vi "Keysight DAQ970-Example2.vi"() -> ()   [LabVIEW 2020, in "Keysight DAQ970.lvlib"]
doc: "This Example initializes the driver, reads a few Identity attributes, Reads Monitor Data ,Read Scan Data and checks the instrument error queue. ."
uses:
  Keysight DAQ970.lvlib
panel:
  out "Display Details":string
  out "Info":T1
  out "Simulate":bool
  in  "Simulate":bool=TRUE
  in  "Select ?":bool=TRUE
  in  "Resource String":string="DAQ2"
  in  "Options String":string="DriverSetup= "
  # "Keysight DAQ970 - Example 2"
  # "------------------------------------------------------------------------------------------------------------------------------------------------------------------------------------------------------------------------"
  # "© Keysight Technologies  2020 - 2021"
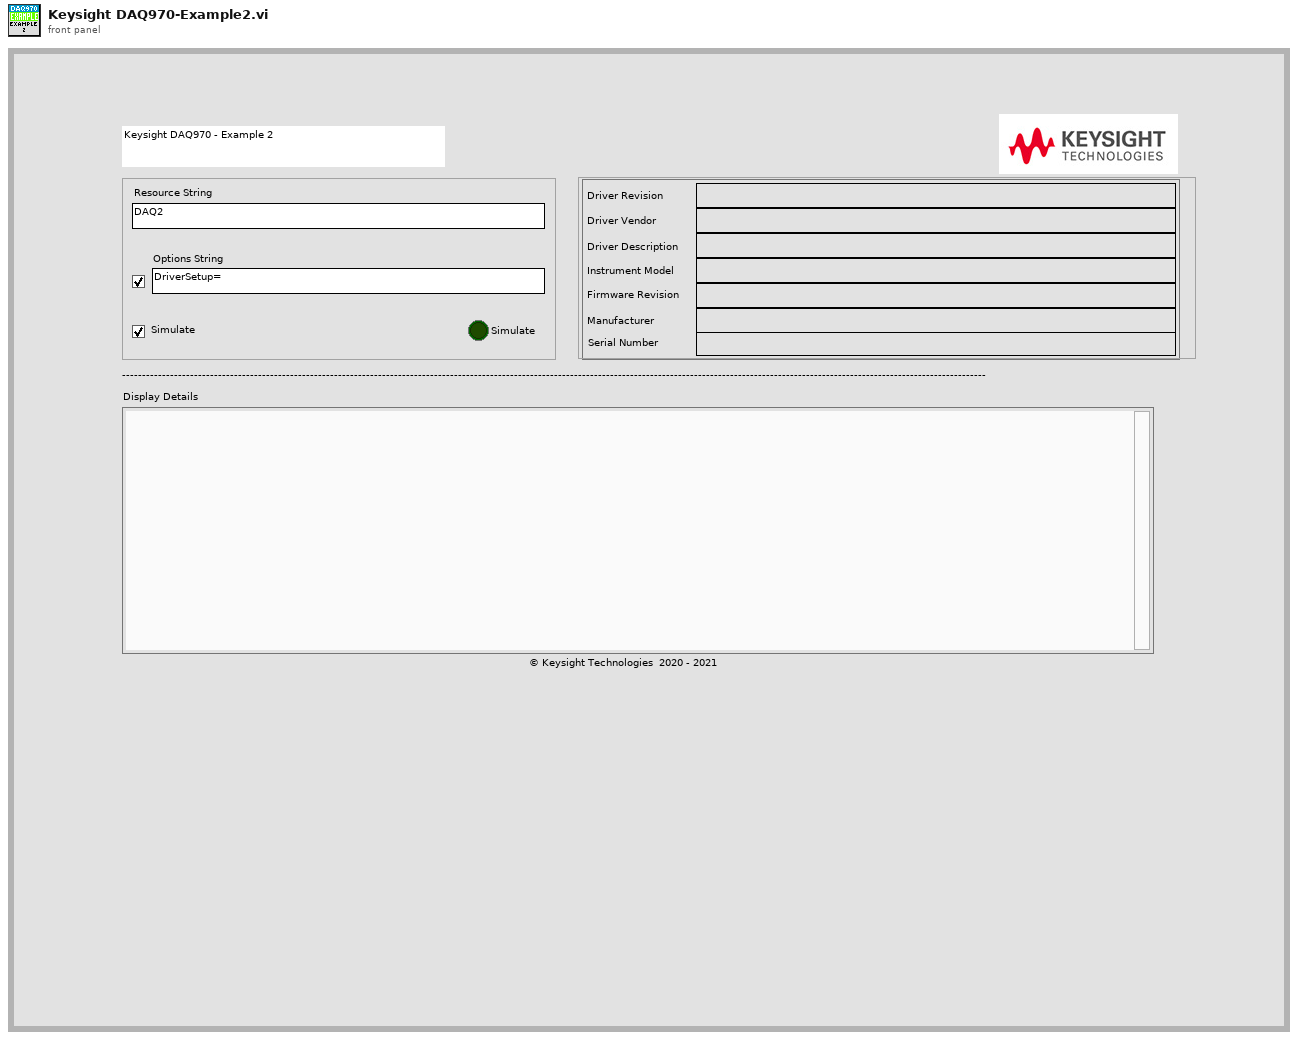
[diagram p1: front panel]
types:
  T1 = cluster{"Driver Revision":string, "Driver Vendor":string, "Driver Description":string, "Instrument Model":string, "Firmware Revision":string, "Instrument Model 2":string, "Firmware Revision 2":string}
  T2 = cluster{"[0]":string, "[1]":string, "[2]":string, "[3]":string, "[4]":string, "[5]":string, "[6]":string}
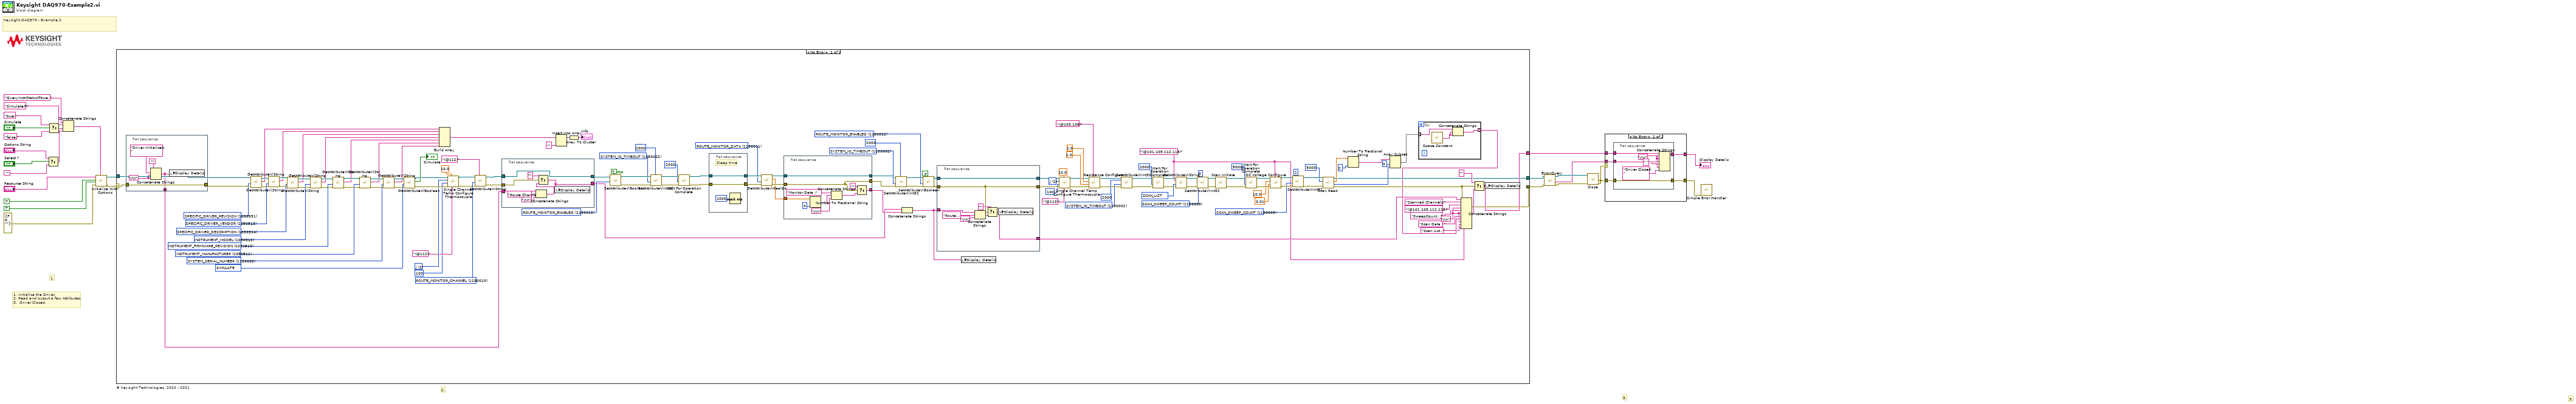
[diagram p0: block diagram]
diagram:
  # "2."
  # "3."
  # "3."
  # "1."
  # "1. Initialize the Driver.\n2. Read and output a few Attributes.\n3.  Driver Closed."
  # "© Keysight Technologies  2020 - 2021"
  # "Keysight DAQ970 - Example 2"
  n1 = Select(t="Options String", s="Select ?", f="") -> (s? t:f=w23:string)
  n2 = Select(t="true,", s="Simulate", f="false,") -> (s? t:f=w25:string)
  n3 = Concatenate Strings("QueryInstrStatus=true, " ("string"), "Simulate=" ("string"), w25, w23) -> (w7:string)
  n4 = call "Initialize With Options.vi"("option string"=w7, "error in (no error)"=errorcluster {"status"=FALSE, "code"=0, "source"=""}, "reset device (Off)"=TRUE, "id query (Off)"=TRUE, "resource string"="Resource String") -> ("error out"=w13:errorcluster, "instrument handle out"=w12:refnum<k15>)  [unwired: 5 in]
  n5 = case shown="No Error" w13 {
    selector: w13 -> [w168 w207]
    tunnel: [w37 w207] -> w3
    tunnel: w12 -> [w139 w206]
    tunnel: [w38 w206] -> w5
    tunnel: [w39 _] -> w15
    frame No Error {
      w27 = "\r\n"
      w51 = u32 1150008 items=["ALARM_MODE"=1150006, "ALARM_SLOPE"=1150007, "FORMAT_TIME_MODE"=1150026, "ROUTE_MONITOR_VIEW"=1150068, "SCAN_CHANNEL_ADVANCE_SOURCE"=1150028, "SCAN_READING_THRESHOLD"=1150031, "SCAN_SINGLE_CHANNEL_SAMPLE_COUNT_PRE_TRIGGER"=1150063, "SCAN_SINGLE_CHANNEL_SAMPLE_COUNT"=1150062, "SCAN_SWEEP_COUNT"=1150008, "SCAN_TRIGGER_OUTPUT_SLOPE"=1150067, "SCAN_TRIGGER_SLOPE"=1150061, "SCAN_TRIGGER_SOURCE"=1150009, "STATUS_ALARM_ENABLE_REGISTER"=1150040, "STATUS_OPERATION_ENABLE_REGISTER"=1150044, "STATUS_QUESTIONABLE_ENABLE_REGISTER"=1150045, "STATUS_SERVICE_REQUEST_ENABLE_REGISTER"=1150047, "STATUS_STANDARD_EVENT_ENABLE_REGISTER"=1150046, "SYSTEM_AUTOCALIBRATION_MONTHLY_INTERVAL_DAY"=1150049, "SYSTEM_AUTOCALIBRATION_OCCURENCE_INTERVAL"=1150048, "SYSTEM_AUTOCALIBRATION_WEEKLY_INTERVAL_DAY"=1150050, "SYSTEM_IO_TIMEOUT"=1150002, "SYSTEM_TRACING_LEVEL"=1150043, "USB_MEMORY_COLUMN_HEADER"=1150054, "USB_MEMORY_COLUMN_SEPARATOR"=1150035, "USB_MEMORY_ROW_LIMIT_COUNT"=1150055] ("AttributeID")
      w128 = 2 items=["b", "g", "j", "k", "n", "r", "s", "t", "def"] ("Type (b)")
      w63 = u32 1150008 items=["ALARM_MODE"=1150006, "ALARM_SLOPE"=1150007, "FORMAT_TIME_MODE"=1150026, "ROUTE_MONITOR_VIEW"=1150068, "SCAN_CHANNEL_ADVANCE_SOURCE"=1150028, "SCAN_READING_THRESHOLD"=1150031, "SCAN_SINGLE_CHANNEL_SAMPLE_COUNT_PRE_TRIGGER"=1150063, "SCAN_SINGLE_CHANNEL_SAMPLE_COUNT"=1150062, "SCAN_SWEEP_COUNT"=1150008, "SCAN_TRIGGER_OUTPUT_SLOPE"=1150067, "SCAN_TRIGGER_SLOPE"=1150061, "SCAN_TRIGGER_SOURCE"=1150009, "STATUS_ALARM_ENABLE_REGISTER"=1150040, "STATUS_OPERATION_ENABLE_REGISTER"=1150044, "STATUS_QUESTIONABLE_ENABLE_REGISTER"=1150045, "STATUS_SERVICE_REQUEST_ENABLE_REGISTER"=1150047, "STATUS_STANDARD_EVENT_ENABLE_REGISTER"=1150046, "SYSTEM_AUTOCALIBRATION_MONTHLY_INTERVAL_DAY"=1150049, "SYSTEM_AUTOCALIBRATION_OCCURENCE_INTERVAL"=1150048, "SYSTEM_AUTOCALIBRATION_WEEKLY_INTERVAL_DAY"=1150050, "SYSTEM_IO_TIMEOUT"=1150002, "SYSTEM_TRACING_LEVEL"=1150043, "USB_MEMORY_COLUMN_HEADER"=1150054, "USB_MEMORY_COLUMN_SEPARATOR"=1150035, "USB_MEMORY_ROW_LIMIT_COUNT"=1150055] ("AttributeID")
      w76 = u32 1150002 items=["ALARM_MODE"=1150006, "ALARM_SLOPE"=1150007, "FORMAT_TIME_MODE"=1150026, "ROUTE_MONITOR_VIEW"=1150068, "SCAN_CHANNEL_ADVANCE_SOURCE"=1150028, "SCAN_READING_THRESHOLD"=1150031, "SCAN_SINGLE_CHANNEL_SAMPLE_COUNT_PRE_TRIGGER"=1150063, "SCAN_SINGLE_CHANNEL_SAMPLE_COUNT"=1150062, "SCAN_SWEEP_COUNT"=1150008, "SCAN_TRIGGER_OUTPUT_SLOPE"=1150067, "SCAN_TRIGGER_SLOPE"=1150061, "SCAN_TRIGGER_SOURCE"=1150009, "STATUS_ALARM_ENABLE_REGISTER"=1150040, "STATUS_OPERATION_ENABLE_REGISTER"=1150044, "STATUS_QUESTIONABLE_ENABLE_REGISTER"=1150045, "STATUS_SERVICE_REQUEST_ENABLE_REGISTER"=1150047, "STATUS_STANDARD_EVENT_ENABLE_REGISTER"=1150046, "SYSTEM_AUTOCALIBRATION_MONTHLY_INTERVAL_DAY"=1150049, "SYSTEM_AUTOCALIBRATION_OCCURENCE_INTERVAL"=1150048, "SYSTEM_AUTOCALIBRATION_WEEKLY_INTERVAL_DAY"=1150050, "SYSTEM_IO_TIMEOUT"=1150002, "SYSTEM_TRACING_LEVEL"=1150043, "USB_MEMORY_COLUMN_HEADER"=1150054, "USB_MEMORY_COLUMN_SEPARATOR"=1150035, "USB_MEMORY_ROW_LIMIT_COUNT"=1150055] ("AttributeID")
      w81 = 2 items=["B", "E", "J", "K", "N", "r", "S", "T"] ("ThermocoupleType (B)")
      w88 = u32 1150012 items=["DISPLAY_ENABLED"=1150016, "FORMAT_ALARM_ENABLED"=1150023, "FORMAT_CHANNEL_ENABLED"=1150024, "FORMAT_TIME_ENABLED"=1150025, "FORMAT_UNITS_ENABLED"=1150027, "ROUTE_MONITOR_ENABLED"=1150012, "SIMULATE"=1050005, "SYSTEM_DMM_ENABLED"=1150018, "SYSTEM_INSTRUMENT_STATE_POWER_ON_RECALL_ENABLED"=1150033, "SYSTEM_LXI_IDENTIFY_ENABLED"=1150032, "SYSTEM_TRACING_ENABLED"=1150041, "USB_MEMORY_LOGGING_ENABLED"=1150034, "USB_MEMORY_MEASUREMENT_DATA_AUTO_SAVE_ENABLED"=1150057, "USB_MEMORY_RECALL_AUTO_ENABLED"=1150052, "USB_MEMORY_ROW_LIMIT_ENABLED"=1150036] ("AttributeID")
      w93 = u32 1150002 items=["ALARM_MODE"=1150006, "ALARM_SLOPE"=1150007, "FORMAT_TIME_MODE"=1150026, "ROUTE_MONITOR_VIEW"=1150068, "SCAN_CHANNEL_ADVANCE_SOURCE"=1150028, "SCAN_READING_THRESHOLD"=1150031, "SCAN_SINGLE_CHANNEL_SAMPLE_COUNT_PRE_TRIGGER"=1150063, "SCAN_SINGLE_CHANNEL_SAMPLE_COUNT"=1150062, "SCAN_SWEEP_COUNT"=1150008, "SCAN_TRIGGER_OUTPUT_SLOPE"=1150067, "SCAN_TRIGGER_SLOPE"=1150061, "SCAN_TRIGGER_SOURCE"=1150009, "STATUS_ALARM_ENABLE_REGISTER"=1150040, "STATUS_OPERATION_ENABLE_REGISTER"=1150044, "STATUS_QUESTIONABLE_ENABLE_REGISTER"=1150045, "STATUS_SERVICE_REQUEST_ENABLE_REGISTER"=1150047, "STATUS_STANDARD_EVENT_ENABLE_REGISTER"=1150046, "SYSTEM_AUTOCALIBRATION_MONTHLY_INTERVAL_DAY"=1150049, "SYSTEM_AUTOCALIBRATION_OCCURENCE_INTERVAL"=1150048, "SYSTEM_AUTOCALIBRATION_WEEKLY_INTERVAL_DAY"=1150050, "SYSTEM_IO_TIMEOUT"=1150002, "SYSTEM_TRACING_LEVEL"=1150043, "USB_MEMORY_COLUMN_HEADER"=1150054, "USB_MEMORY_COLUMN_SEPARATOR"=1150035, "USB_MEMORY_ROW_LIMIT_COUNT"=1150055] ("AttributeID")
      w98 = u32 1150011 items=["ROUTE_MONITOR_DATA"=1150011, "ROUTE_MONITOR_FULL_DATA"=1150069, "SCAN_SINGLE_CHANNEL_SAMPLE_INTERVAL"=1150064, "SCAN_TIMER_INTERVAL"=1150029, "SCAN_TRIGGER_DELAY"=1150059, "SCAN_TRIGGER_LEVEL"=1150060, "SYSTEM_LINE_FREQUENCY"=1150037] ("AttributeID")
      w107 = u32 1150002 items=["ALARM_MODE"=1150006, "ALARM_SLOPE"=1150007, "FORMAT_TIME_MODE"=1150026, "ROUTE_MONITOR_VIEW"=1150068, "SCAN_CHANNEL_ADVANCE_SOURCE"=1150028, "SCAN_READING_THRESHOLD"=1150031, "SCAN_SINGLE_CHANNEL_SAMPLE_COUNT_PRE_TRIGGER"=1150063, "SCAN_SINGLE_CHANNEL_SAMPLE_COUNT"=1150062, "SCAN_SWEEP_COUNT"=1150008, "SCAN_TRIGGER_OUTPUT_SLOPE"=1150067, "SCAN_TRIGGER_SLOPE"=1150061, "SCAN_TRIGGER_SOURCE"=1150009, "STATUS_ALARM_ENABLE_REGISTER"=1150040, "STATUS_OPERATION_ENABLE_REGISTER"=1150044, "STATUS_QUESTIONABLE_ENABLE_REGISTER"=1150045, "STATUS_SERVICE_REQUEST_ENABLE_REGISTER"=1150047, "STATUS_STANDARD_EVENT_ENABLE_REGISTER"=1150046, "SYSTEM_AUTOCALIBRATION_MONTHLY_INTERVAL_DAY"=1150049, "SYSTEM_AUTOCALIBRATION_OCCURENCE_INTERVAL"=1150048, "SYSTEM_AUTOCALIBRATION_WEEKLY_INTERVAL_DAY"=1150050, "SYSTEM_IO_TIMEOUT"=1150002, "SYSTEM_TRACING_LEVEL"=1150043, "USB_MEMORY_COLUMN_HEADER"=1150054, "USB_MEMORY_COLUMN_SEPARATOR"=1150035, "USB_MEMORY_ROW_LIMIT_COUNT"=1150055] ("AttributeID")
      w117 = u32 1150010 items=["CALIBRATION_MESSAGE"=1150015, "DISPLAY_TEXT"=1150017, "ROUTE_MONITOR_CHANNEL"=1150010, "SCAN_LIST"=1150004, "SYSTEM_DATE"=1150020, "SYSTEM_TIME"=1150021, "SYSTEM_TRACING_FILE_NAME"=1150042, "USB_MEMORY_DATA_FILE"=1150056, "USB_MEMORY_MEASUREMENTS_DATA_AUTO_SAVE_FILE"=1150058, "USB_MEMORY_SELECT_RECALL_AUTO_FILE"=1150053] ("AttributeID")
      w120 = u32 1150012 items=["DISPLAY_ENABLED"=1150016, "FORMAT_ALARM_ENABLED"=1150023, "FORMAT_CHANNEL_ENABLED"=1150024, "FORMAT_TIME_ENABLED"=1150025, "FORMAT_UNITS_ENABLED"=1150027, "ROUTE_MONITOR_ENABLED"=1150012, "SIMULATE"=1050005, "SYSTEM_DMM_ENABLED"=1150018, "SYSTEM_INSTRUMENT_STATE_POWER_ON_RECALL_ENABLED"=1150033, "SYSTEM_LXI_IDENTIFY_ENABLED"=1150032, "SYSTEM_TRACING_ENABLED"=1150041, "USB_MEMORY_LOGGING_ENABLED"=1150034, "USB_MEMORY_MEASUREMENT_DATA_AUTO_SAVE_ENABLED"=1150057, "USB_MEMORY_RECALL_AUTO_ENABLED"=1150052, "USB_MEMORY_ROW_LIMIT_ENABLED"=1150036] ("AttributeID")
      w121 = u32 1150004 items=["CALIBRATION_MESSAGE"=1150015, "DISPLAY_TEXT"=1150017, "ROUTE_MONITOR_CHANNEL"=1150010, "SCAN_LIST"=1150004, "SYSTEM_DATE"=1150020, "SYSTEM_TIME"=1150021, "SYSTEM_TRACING_FILE_NAME"=1150042, "USB_MEMORY_DATA_FILE"=1150056, "USB_MEMORY_MEASUREMENTS_DATA_AUTO_SAVE_FILE"=1150058, "USB_MEMORY_SELECT_RECALL_AUTO_FILE"=1150053] ("AttributeID")
      w162 = u32 1050005 items=["DISPLAY_ENABLED"=1150016, "FORMAT_ALARM_ENABLED"=1150023, "FORMAT_CHANNEL_ENABLED"=1150024, "FORMAT_TIME_ENABLED"=1150025, "FORMAT_UNITS_ENABLED"=1150027, "ROUTE_MONITOR_ENABLED"=1150012, "SIMULATE"=1050005, "SYSTEM_AUTOCALIBRATION_GET_ALL_MODULE_STATE"=1150051, "SYSTEM_DMM_ENABLED"=1150018, "SYSTEM_DMM_INSTALLED"=1150019, "SYSTEM_INSTRUMENT_STATE_POWER_ON_RECALL_ENABLED"=1150033, "SYSTEM_LXI_IDENTIFY_ENABLED"=1150032, "SYSTEM_TRACING_ENABLED"=1150041, "USB_MEMORY_LOGGING_ENABLED"=1150034, "USB_MEMORY_MEASUREMENT_DATA_AUTO_SAVE_ENABLED"=1150057, "USB_MEMORY_RECALL_AUTO_ENABLED"=1150052, "USB_MEMORY_ROW_LIMIT_ENABLED"=1150036] ("AttributeID")
      w161 = u32 1150003 items=["CALIBRATION_DATE"=1150065, "CALIBRATION_MESSAGE"=1150015, "CALIBRATION_TIME"=1150066, "DISPLAY_TEXT"=1150017, "DRIVER_SETUP"=1050007, "GROUP_CAPABILITIES"=1050401, "INSTRUMENT_FIRMWARE_REVISION"=1050510, "INSTRUMENT_MANUFACTURER"=1050511, "INSTRUMENT_MODEL"=1050512, "IO_RESOURCE_DESCRIPTOR"=1050304, "LOGICAL_NAME"=1050305, "ROUTE_MONITOR_CHANNEL"=1150010, "SCAN_LIST"=1150004, "SCAN_STARTTIME"=1150022, "SPECIFIC_DRIVER_DESCRIPTION"=1050514, "SPECIFIC_DRIVER_PREFIX"=1050302, "SPECIFIC_DRIVER_REVISION"=1050551, "SPECIFIC_DRIVER_VENDOR"=1050513, "SUPPORTED_INSTRUMENT_MODELS"=1050327, "SYSTEM_DATE"=1150020, "SYSTEM_SERIAL_NUMBER"=1150003, "SYSTEM_TIME"=1150021, "SYSTEM_TRACING_FILE_NAME"=1150042, "USB_MEMORY_DATA_FILE"=1150056, "USB_MEMORY_MEASUREMENTS_DATA_AUTO_SAVE_FILE"=1150058, "USB_MEMORY_SELECT_RECALL_AUTO_FILE"=1150053] ("AttributeID")
      w160 = u32 1050511 items=["CALIBRATION_DATE"=1150065, "CALIBRATION_MESSAGE"=1150015, "CALIBRATION_TIME"=1150066, "DISPLAY_TEXT"=1150017, "DRIVER_SETUP"=1050007, "GROUP_CAPABILITIES"=1050401, "INSTRUMENT_FIRMWARE_REVISION"=1050510, "INSTRUMENT_MANUFACTURER"=1050511, "INSTRUMENT_MODEL"=1050512, "IO_RESOURCE_DESCRIPTOR"=1050304, "LOGICAL_NAME"=1050305, "ROUTE_MONITOR_CHANNEL"=1150010, "SCAN_LIST"=1150004, "SCAN_STARTTIME"=1150022, "SPECIFIC_DRIVER_DESCRIPTION"=1050514, "SPECIFIC_DRIVER_PREFIX"=1050302, "SPECIFIC_DRIVER_REVISION"=1050551, "SPECIFIC_DRIVER_VENDOR"=1050513, "SUPPORTED_INSTRUMENT_MODELS"=1050327, "SYSTEM_DATE"=1150020, "SYSTEM_SERIAL_NUMBER"=1150003, "SYSTEM_TIME"=1150021, "SYSTEM_TRACING_FILE_NAME"=1150042, "USB_MEMORY_DATA_FILE"=1150056, "USB_MEMORY_MEASUREMENTS_DATA_AUTO_SAVE_FILE"=1150058, "USB_MEMORY_SELECT_RECALL_AUTO_FILE"=1150053] ("AttributeID")
      w159 = u32 1050510 items=["CALIBRATION_DATE"=1150065, "CALIBRATION_MESSAGE"=1150015, "CALIBRATION_TIME"=1150066, "DISPLAY_TEXT"=1150017, "DRIVER_SETUP"=1050007, "GROUP_CAPABILITIES"=1050401, "INSTRUMENT_FIRMWARE_REVISION"=1050510, "INSTRUMENT_MANUFACTURER"=1050511, "INSTRUMENT_MODEL"=1050512, "IO_RESOURCE_DESCRIPTOR"=1050304, "LOGICAL_NAME"=1050305, "ROUTE_MONITOR_CHANNEL"=1150010, "SCAN_LIST"=1150004, "SCAN_STARTTIME"=1150022, "SPECIFIC_DRIVER_DESCRIPTION"=1050514, "SPECIFIC_DRIVER_PREFIX"=1050302, "SPECIFIC_DRIVER_REVISION"=1050551, "SPECIFIC_DRIVER_VENDOR"=1050513, "SUPPORTED_INSTRUMENT_MODELS"=1050327, "SYSTEM_DATE"=1150020, "SYSTEM_SERIAL_NUMBER"=1150003, "SYSTEM_TIME"=1150021, "SYSTEM_TRACING_FILE_NAME"=1150042, "USB_MEMORY_DATA_FILE"=1150056, "USB_MEMORY_MEASUREMENTS_DATA_AUTO_SAVE_FILE"=1150058, "USB_MEMORY_SELECT_RECALL_AUTO_FILE"=1150053] ("AttributeID")
      w158 = u32 1050512 items=["CALIBRATION_DATE"=1150065, "CALIBRATION_MESSAGE"=1150015, "CALIBRATION_TIME"=1150066, "DISPLAY_TEXT"=1150017, "DRIVER_SETUP"=1050007, "GROUP_CAPABILITIES"=1050401, "INSTRUMENT_FIRMWARE_REVISION"=1050510, "INSTRUMENT_MANUFACTURER"=1050511, "INSTRUMENT_MODEL"=1050512, "IO_RESOURCE_DESCRIPTOR"=1050304, "LOGICAL_NAME"=1050305, "ROUTE_MONITOR_CHANNEL"=1150010, "SCAN_LIST"=1150004, "SCAN_STARTTIME"=1150022, "SPECIFIC_DRIVER_DESCRIPTION"=1050514, "SPECIFIC_DRIVER_PREFIX"=1050302, "SPECIFIC_DRIVER_REVISION"=1050551, "SPECIFIC_DRIVER_VENDOR"=1050513, "SUPPORTED_INSTRUMENT_MODELS"=1050327, "SYSTEM_DATE"=1150020, "SYSTEM_SERIAL_NUMBER"=1150003, "SYSTEM_TIME"=1150021, "SYSTEM_TRACING_FILE_NAME"=1150042, "USB_MEMORY_DATA_FILE"=1150056, "USB_MEMORY_MEASUREMENTS_DATA_AUTO_SAVE_FILE"=1150058, "USB_MEMORY_SELECT_RECALL_AUTO_FILE"=1150053] ("AttributeID")
      w157 = u32 1050514 items=["CALIBRATION_DATE"=1150065, "CALIBRATION_MESSAGE"=1150015, "CALIBRATION_TIME"=1150066, "DISPLAY_TEXT"=1150017, "DRIVER_SETUP"=1050007, "GROUP_CAPABILITIES"=1050401, "INSTRUMENT_FIRMWARE_REVISION"=1050510, "INSTRUMENT_MANUFACTURER"=1050511, "INSTRUMENT_MODEL"=1050512, "IO_RESOURCE_DESCRIPTOR"=1050304, "LOGICAL_NAME"=1050305, "ROUTE_MONITOR_CHANNEL"=1150010, "SCAN_LIST"=1150004, "SCAN_STARTTIME"=1150022, "SPECIFIC_DRIVER_DESCRIPTION"=1050514, "SPECIFIC_DRIVER_PREFIX"=1050302, "SPECIFIC_DRIVER_REVISION"=1050551, "SPECIFIC_DRIVER_VENDOR"=1050513, "SUPPORTED_INSTRUMENT_MODELS"=1050327, "SYSTEM_DATE"=1150020, "SYSTEM_SERIAL_NUMBER"=1150003, "SYSTEM_TIME"=1150021, "SYSTEM_TRACING_FILE_NAME"=1150042, "USB_MEMORY_DATA_FILE"=1150056, "USB_MEMORY_MEASUREMENTS_DATA_AUTO_SAVE_FILE"=1150058, "USB_MEMORY_SELECT_RECALL_AUTO_FILE"=1150053] ("AttributeID")
      w156 = u32 1050513 items=["CALIBRATION_DATE"=1150065, "CALIBRATION_MESSAGE"=1150015, "CALIBRATION_TIME"=1150066, "DISPLAY_TEXT"=1150017, "DRIVER_SETUP"=1050007, "GROUP_CAPABILITIES"=1050401, "INSTRUMENT_FIRMWARE_REVISION"=1050510, "INSTRUMENT_MANUFACTURER"=1050511, "INSTRUMENT_MODEL"=1050512, "IO_RESOURCE_DESCRIPTOR"=1050304, "LOGICAL_NAME"=1050305, "ROUTE_MONITOR_CHANNEL"=1150010, "SCAN_LIST"=1150004, "SCAN_STARTTIME"=1150022, "SPECIFIC_DRIVER_DESCRIPTION"=1050514, "SPECIFIC_DRIVER_PREFIX"=1050302, "SPECIFIC_DRIVER_REVISION"=1050551, "SPECIFIC_DRIVER_VENDOR"=1050513, "SUPPORTED_INSTRUMENT_MODELS"=1050327, "SYSTEM_DATE"=1150020, "SYSTEM_SERIAL_NUMBER"=1150003, "SYSTEM_TIME"=1150021, "SYSTEM_TRACING_FILE_NAME"=1150042, "USB_MEMORY_DATA_FILE"=1150056, "USB_MEMORY_MEASUREMENTS_DATA_AUTO_SAVE_FILE"=1150058, "USB_MEMORY_SELECT_RECALL_AUTO_FILE"=1150053] ("AttributeID")
      w155 = u32 1050551 items=["CALIBRATION_DATE"=1150065, "CALIBRATION_MESSAGE"=1150015, "CALIBRATION_TIME"=1150066, "DISPLAY_TEXT"=1150017, "DRIVER_SETUP"=1050007, "GROUP_CAPABILITIES"=1050401, "INSTRUMENT_FIRMWARE_REVISION"=1050510, "INSTRUMENT_MANUFACTURER"=1050511, "INSTRUMENT_MODEL"=1050512, "IO_RESOURCE_DESCRIPTOR"=1050304, "LOGICAL_NAME"=1050305, "ROUTE_MONITOR_CHANNEL"=1150010, "SCAN_LIST"=1150004, "SCAN_STARTTIME"=1150022, "SPECIFIC_DRIVER_DESCRIPTION"=1050514, "SPECIFIC_DRIVER_PREFIX"=1050302, "SPECIFIC_DRIVER_REVISION"=1050551, "SPECIFIC_DRIVER_VENDOR"=1050513, "SUPPORTED_INSTRUMENT_MODELS"=1050327, "SYSTEM_DATE"=1150020, "SYSTEM_SERIAL_NUMBER"=1150003, "SYSTEM_TIME"=1150021, "SYSTEM_TRACING_FILE_NAME"=1150042, "USB_MEMORY_DATA_FILE"=1150056, "USB_MEMORY_MEASUREMENTS_DATA_AUTO_SAVE_FILE"=1150058, "USB_MEMORY_SELECT_RECALL_AUTO_FILE"=1150053] ("AttributeID")
      w29 = "(@101,105,112,113)" ("AttributeValue")
      n6 = flat-sequence {
        tunnel: w168 -> [w205]
        tunnel: [w205] -> w138
        tunnel: [w201] -> w114
        frame #0 {
          w202 = "\r\n"
          n7 = Concatenate Strings("", "Driver Initialized.", w202, w202) -> (w201:string)
          n8 = local write "Display Details"(w201) -> ()
        }
      }
      n9 = call "GetAttributeViString.vi"("error in (no error)"=w138, "AttributeID"=w155, "instrument handle"=w139) -> ("error out"=w141:errorcluster, "AttributeValue"=w137:string, "instrument handle out"=w142:refnum<k15>)  [unwired: 6 in]
      n10 = call "GetAttributeViString.vi"("error in (no error)"=w141, "AttributeID"=w156, "instrument handle"=w142) -> ("error out"=w143:errorcluster, "AttributeValue"=w136:string, "instrument handle out"=w144:refnum<k15>)  [unwired: 6 in]
      n11 = call "GetAttributeViString.vi"("error in (no error)"=w143, "AttributeID"=w157, "instrument handle"=w144) -> ("error out"=w146:errorcluster, "AttributeValue"=w135:string, "instrument handle out"=w145:refnum<k15>)  [unwired: 6 in]
      n12 = call "GetAttributeViString.vi"("error in (no error)"=w146, "AttributeID"=w158, "instrument handle"=w145) -> ("error out"=w147:errorcluster, "AttributeValue"=w134:string, "instrument handle out"=w148:refnum<k15>)  [unwired: 6 in]
      n13 = call "GetAttributeViString.vi"("error in (no error)"=w147, "AttributeID"=w159, "instrument handle"=w148) -> ("error out"=w149:errorcluster, "AttributeValue"=w133:string, "instrument handle out"=w150:refnum<k15>)  [unwired: 6 in]
      n14 = call "GetAttributeViString.vi"("error in (no error)"=w149, "AttributeID"=w160, "instrument handle"=w150) -> ("error out"=w152:errorcluster, "AttributeValue"=w132:string, "instrument handle out"=w151:refnum<k15>)  [unwired: 6 in]
      n15 = call "GetAttributeViString.vi"("error in (no error)"=w152, "AttributeID"=w161, "instrument handle"=w151) -> ("error out"=w154:errorcluster, "AttributeValue"=w131:string, "instrument handle out"=w153:refnum<k15>)  [unwired: 6 in]
      n16 = call "GetAttributeViBoolean.vi"("error in (no error)"=w154, "AttributeID"=w162, "instrument handle"=w153) -> ("error out"=w130:errorcluster, "AttributeValue"=→"Simulate":bool, "instrument handle out"=w129:refnum<k15>)  [unwired: 6 in]
      n17 = Build Array(w137, w136, w135, w134, w133, w132, w131) -> (w165:string[])
      n18 = call "Single Channel Temp Configure Thermocouple.vi"("Channel"="(@112)" ("ChannelList"), "SampTime"=10.0 ("Sample Time"), "error in (no error)"=w130, "SampCount"=100, "ThermocoupleType (B)"=w128, "instrument handle"=w129) -> ("error out"=w116:errorcluster, "instrument handle out"=w118:refnum<k15>)  [unwired: 4 in]
      n19 = call "SetAttributeViString.vi"("AttributeValue"="(@112)", "error in (no error)"=w116, "AttributeID"=w117, "instrument handle"=w118) -> ("error out"=w113:errorcluster, "instrument handle out"=w112:refnum<k15>)  [unwired: 6 in]
      n20 = flat-sequence {
        tunnel: w114 -> [w192]
        tunnel: w113 -> [w188]
        tunnel: [w186] -> w99
        tunnel: [w191] -> w111
        tunnel: w112 -> [w191]
        frame #0 {
          n21 = Concatenate Strings(w192, "Route Channel Monitoring Enabled !!!", "\r\n") -> (w187:string)
          n22 = Select(t="", s=w188, f=w187) -> (s? t:f=w186:string)
          n23 = local write "Display Details"(w186) -> ()
        }
      }
      n24 = Insert Into Array(array=w165, new element="" ("new element/subarray")) -> (w166:string[])  [unwired: 1 in]
      n25 = Array To Cluster(array=w166) -> (cluster=→"Info":T2)
      n26 = call "SetAttributeViBoolean.vi"("AttributeValue (Off)"=TRUE, "AttributeID"=w120, "instrument handle"=w111) -> ("error out"=w109:errorcluster, "instrument handle out"=w110:refnum<k15>)  [unwired: 7 in]
      n27 = call "SetAttributeViInt32.vi"("AttributeValue"=2000, "error in (no error)"=w109, "AttributeID"=w107, "instrument handle"=w110) -> ("error out"=w105:errorcluster, "instrument handle out"=w106:refnum<k15>)  [unwired: 6 in]
      n28 = call "Wait For Operation Complete.vi"("error in (no error)"=w105, "MaxTimeMilliseconds"=2000, "instrument handle"=w106) -> ("error out"=w102:errorcluster, "instrument handle out"=w103:refnum<k15>)  [unwired: 7 in]
      n29 = flat-sequence {
        tunnel: [w183] -> w101
        tunnel: w103 -> [w183]
        tunnel: [w182] -> w100
        tunnel: w102 -> [w182]
        frame #0 {
          # "Sleep time"
          n30 = Wait (ms)(milliseconds to wait=u32 1000) -> ()  [unwired: 1 out]
        }
      }
      n31 = call "GetAttributeViReal64.vi"("error in (no error)"=w100, "AttributeID"=w98, "instrument handle"=w101) -> ("error out"=w97:errorcluster, "AttributeValue"=w36:dbl, "instrument handle out"=w96:refnum<k15>)  [unwired: 6 in]
      n32 = flat-sequence {
        tunnel: w97 -> [w174]
        tunnel: [w176] -> w92
        tunnel: w96 -> [w176]
        tunnel: [w175] -> w95
        tunnel: [w174] -> w91
        tunnel: w36 -> [w173]
        frame #0 {
          n33 = Number To Fractional String(number=w173, precision (6)=i16 0) -> (F-format string=w180:string)  [unwired: 2 in]
          n34 = Concatenate Strings("Monitor Data :", w180, "\r\n") -> (w179:string)
          n35 = Select(t="", s=w174, f=w179) -> (s? t:f=w175:string)
        }
      }
      n36 = call "SetAttributeViInt32.vi"("AttributeValue"=2000, "error in (no error)"=w91, "AttributeID"=w93, "instrument handle"=w92) -> ("error out"=w89:errorcluster, "instrument handle out"=w90:refnum<k15>)  [unwired: 6 in]
      n37 = Concatenate Strings(w99, w95) -> (w164:string)
      n38 = call "SetAttributeViBoolean.vi"("AttributeValue (Off)"=FALSE, "error in (no error)"=w89, "AttributeID"=w88, "instrument handle"=w90) -> ("error out"=w85:errorcluster, "instrument handle out"=w86:refnum<k15>)  [unwired: 6 in]
      n39 = flat-sequence {
        tunnel: [w193] -> w83
        tunnel: w164 -> [w200]
        tunnel: [w196] -> w40
        tunnel: [w194] -> w84
        tunnel: w86 -> [w194]
        tunnel: w85 -> [w193]
        frame #0 {
          n40 = Concatenate Strings(w200, "Route Channel Monitoring Disabled !!!", "\r\n") -> (w197:string)
          n41 = Select(t="", s=w193, f=w197) -> (s? t:f=w196:string)
          n42 = local write "Display Details"(w196) -> ()
        }
      }
      n43 = local write "Display Details"(w164) -> ()
      n44 = call "Single Channel Temp Configure Thermocouple.vi"("Channel"="(@113)", "SampTime"=10.0, "error in (no error)"=w83, "SampCount"=100, "ThermocoupleType (B)"=w81, "instrument handle"=w84) -> ("error out"=w77:errorcluster, "instrument handle out"=w78:refnum<k15>)  [unwired: 4 in]
      n45 = call "Resistance Configure.vi"("ChannelList"="(@103,108)", "error in (no error)"=w77, "Resolution"=1.0, "Range"=1.0, "instrument handle"=w78) -> ("error out"=w74:errorcluster, "instrument handle out"=w73:refnum<k15>)  [unwired: 5 in]
      n46 = call "SetAttributeViInt32.vi"("AttributeValue"=2000, "error in (no error)"=w74, "AttributeID"=w76, "instrument handle"=w73) -> ("error out"=w70:errorcluster, "instrument handle out"=w71:refnum<k15>)  [unwired: 6 in]
      n47 = call "Wait For Operation Complete.vi"("error in (no error)"=w70, "MaxTimeMilliseconds"=2000, "instrument handle"=w71) -> ("error out"=w69:errorcluster, "instrument handle out"=w68:refnum<k15>)  [unwired: 7 in]
      n48 = call "SetAttributeViString.vi"("AttributeValue"=w29, "error in (no error)"=w69, "AttributeID"=w121, "instrument handle"=w68) -> ("error out"=w66:errorcluster, "instrument handle out"=w67:refnum<k15>)  [unwired: 6 in]
      n49 = call "SetAttributeViInt32.vi"("AttributeValue"=5, "error in (no error)"=w66, "AttributeID"=w63, "instrument handle"=w67) -> ("error out"=w64:errorcluster, "instrument handle out"=w65:refnum<k15>)  [unwired: 6 in]
      n50 = call "Scan Initiate.vi"("error in (no error)"=w64, "instrument handle"=w65) -> ("error out"=w59:errorcluster, "instrument handle out"=w60:refnum<k15>)  [unwired: 8 in]
      n51 = call "Wait For Operation Complete.vi"("error in (no error)"=w59, "MaxTimeMilliseconds"=5000, "instrument handle"=w60) -> ("error out"=w57:errorcluster, "instrument handle out"=w58:refnum<k15>)  [unwired: 7 in]
      n52 = call "DC Voltage Configure.vi"("ChannelList"=w29, "error in (no error)"=w57, "Resolution"=0.01, "Range"=10.0, "instrument handle"=w58) -> ("error out"=w53:errorcluster, "instrument handle out"=w52:refnum<k15>)  [unwired: 5 in]
      n53 = call "SetAttributeViInt32.vi"("AttributeValue"=2, "error in (no error)"=w53, "AttributeID"=w51, "instrument handle"=w52) -> ("error out"=w50:errorcluster, "instrument handle out"=w49:refnum<k15>)  [unwired: 6 in]
      n54 = call "Scan Read.vi"("error in (no error)"=w50, "MaxTimeMilliseconds"=5000, "instrument handle"=w49) -> ("error out"=w37:errorcluster, "ValActualSize"=w33:i32, "Val"=w47:dbl[], "instrument handle out"=w38:refnum<k15>)  [unwired: 5 in]
      n55 = Number To Fractional String(number=w47, precision (6)=i16 2) -> (F-format string=w35:string[])  [unwired: 2 in]
      n56 = Array Subset(array=w35, index=0, length=w33) -> (w31:string[])
      n57 = for {
        tunnel: w31 -> [w171] mode=indexing
        tunnel: [w170] -> w30 mode=indexing
        n58 = call <vilib>:"Space Constant.vi"() -> ("String"=w169:string)
        n59 = Concatenate Strings(w171, w169, w169) -> (w170:string)
      }
      n60 = Concatenate Strings(w40, "Scanned Channels:" ("t"), "(@101,105,112,113)" ("AttributeValue"), w27, "SweepCount : 2" ("t"), w27, "Scan Data : " ("t"), w30, w27, "Scan List : " ("t"), w29) -> (w45:string)
      n61 = Select(t="", s=w37, f=w45) -> (s? t:f=w39:string)
      n62 = local write "Display Details"(w39) -> ()
    }
    frame Error {
    }
  }
  n63 = call "Error-Query.vi"("error in (no error)"=w3, "instrument handle"=w5) -> ("error out"=w2:errorcluster, "error message"=w1:string, "instrument handle out"=w4:refnum<k15>)  [unwired: 6 in, 1 out]
  n64 = call "Close.vi"("error in (no error)"=w2, "instrument handle"=w4) -> ("error out"=w6:errorcluster)  [unwired: 9 in]
  n65 = case shown="No Error" w6 {
    tunnel: w6 -> [w212 w220]
    tunnel: [w211 w220] -> w16
    tunnel: w15 -> [w210 w221]
    tunnel: [w209 w221] -> w14
    tunnel: w1 -> [w208 _]
    frame No Error {
      n66 = flat-sequence {
        tunnel: w212 -> [w219]
        tunnel: [w219] -> w211
        tunnel: w210 -> [w218]
        tunnel: [w217] -> w209
        tunnel: w208 -> [w215]
        frame #0 {
          w213 = "\r\n"
          n67 = Concatenate Strings(w218, w213, w213, w215, "." ("string"), w213, "Driver Closed.") -> (w217:string)
        }
      }
    }
    frame Error {
    }
  }
  "Display Details" <- w14
  n68 = call <vilib>:"Simple Error Handler.vi"("error in (no error)"=w16) -> ()  [unwired: 4 in, 5 out]
